vi "Find Downstream Terms.vi"(6 "Distances":dbl[](array[numeric]), 8 "Error":errorcluster, 9 "Segment Descriptors":T1[](array[typedef]) {"Direction" items=["Up", "Down", "Left", "Right"]}, 10 "Terminal Joint Indices":i32[](array[numeric]), 11 "Wire Refnum":refnum<vi>) -> (0 "Error Out":errorcluster, 1 "Array Out":refnum<vi>[](array[refnum]), 2 "Source Node Out":refnum<vi>, 3 "Wire Refnum Out":refnum<vi>)   [LabVIEW 2012, in "Scripting Tools.lvlib"]
doc: "Given an array of wire segment descriptors, an array of terminal joints and an array of distances to an arbitary point, figures out which segment is nearest and then returns all the downstream terminals."
uses:
  Scripting Tools.lvlib
  Wire Segment Descriptor Type.ctl
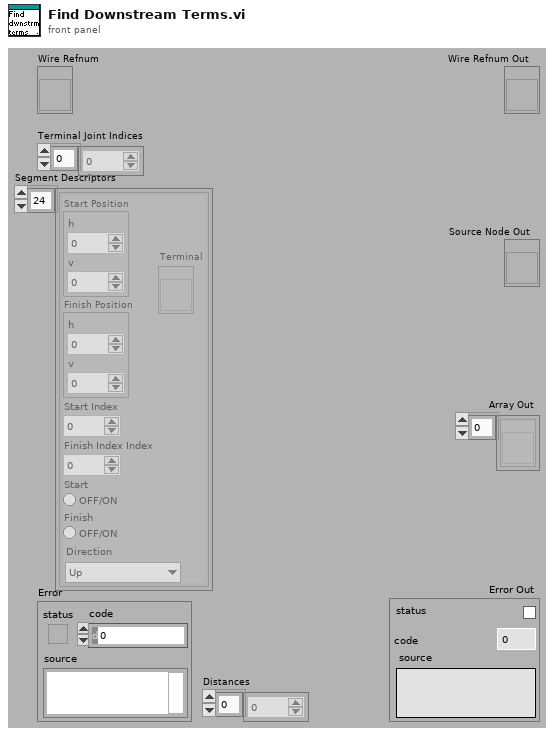
[diagram p1: front panel]
types:
  T1 = typedef "Scripting Tools.lvlib/Wire Segment Descriptor Type.ctl" = cluster{"Start Position":cluster{"h":i16, "v":i16}, "Finish Position":cluster{"h":i16, "v":i16}, "Start Index":i32, "Finish Index Index":i32, "Start":bool, "Finish":bool, "Direction":u16, "Terminal":refnum<vi>}
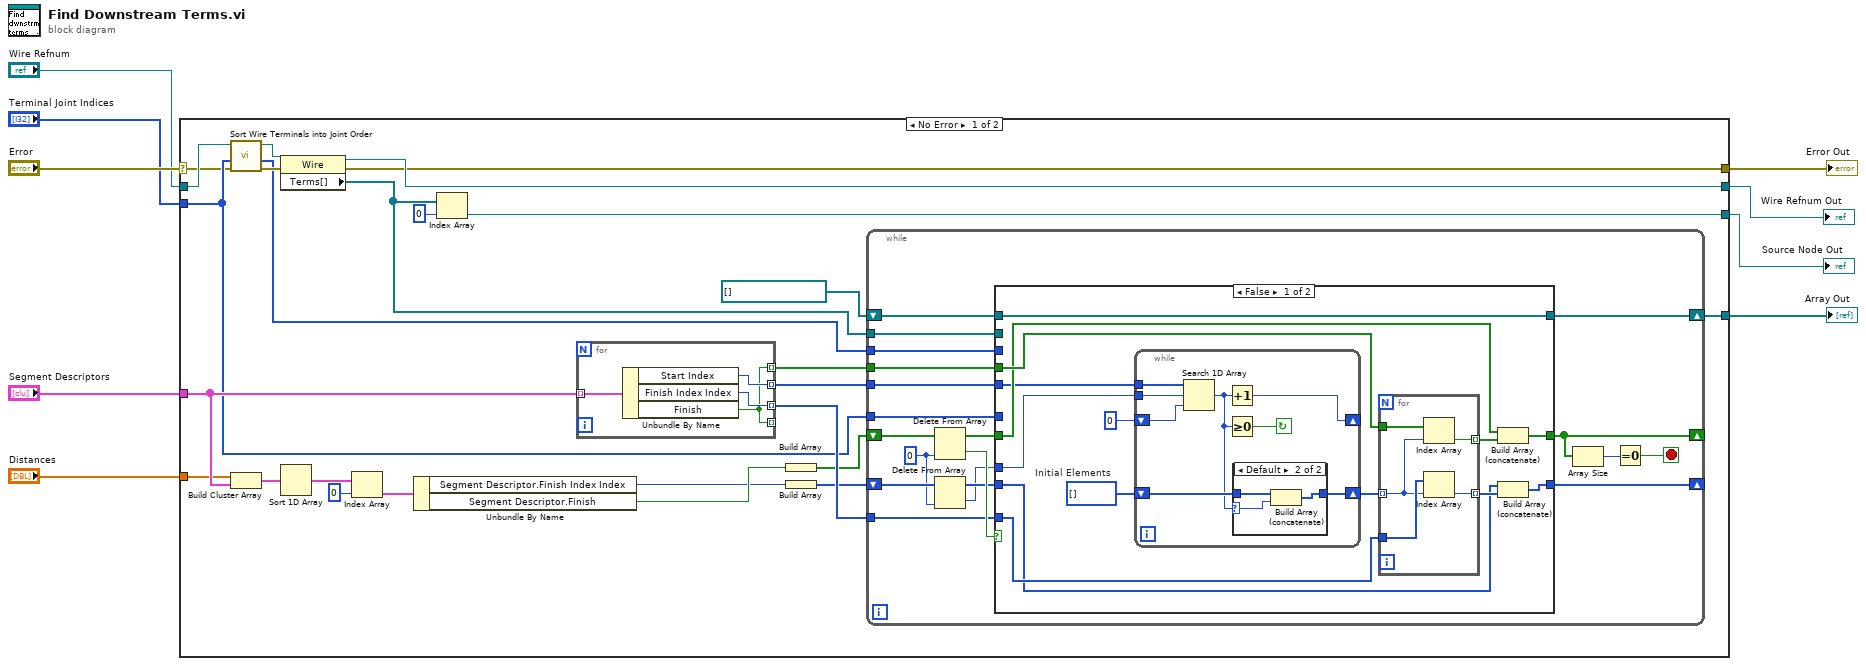
[diagram p0: block diagram]
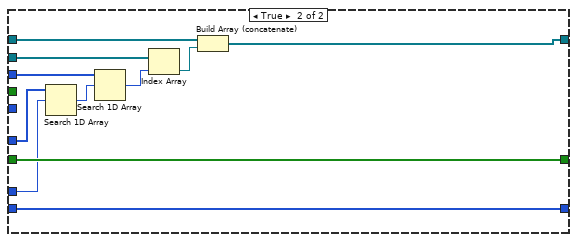
[diagram p3: hidden frame]
diagram:
  n1 = case shown="No Error" "Error" {
    selector: "Error" -> [w10 w102]
    tunnel: [w18 w101] -> w9
    tunnel: [w17 w102] -> w8
    tunnel: "Wire Refnum" -> [w15 w101]
    tunnel: [w34 _] -> w5
    tunnel: [w33 _] -> w4
    tunnel: "Segment Descriptors" -> [w24 _]
    tunnel: "Distances" -> [w19 _]
    tunnel: "Terminal Joint Indices" -> [w12 _]
    frame No Error {
      n2 = call "Sort Wire Terminals into Joint Order.vi"("Error IO"=w10, "Terminal Joint Indices"=w12, "Wire Refnum"=w15) -> ("Error Out"=w13:errorcluster, "Sorted Pointers Out"=w11:i32[], "Wire Refnum Out"=w14:refnum<vi>)  [unwired: 4 in, 2 out]
      n3 = Build Cluster Array(w19, w24) -> (w20:cluster{"d":dbl, "Segment Descriptor":T1}[])
      n4 = property class="Wire"(reference=w14, error in=w13) -> (reference out=w18:refnum<vi>, error out=w17:errorcluster, "Terms[]"=w16:refnum<vi>[])
      n5 = Sort 1D Array(array=w20) -> (sorted array=w21:cluster{"d":dbl, "Segment Descriptor":T1}[])
      n6 = Index Array(array=w21, index=0) -> (element=w23:cluster{"d":dbl, "Segment Descriptor":T1})
      n7 = Unbundle By Name(w23) -> ("Segment Descriptor.Finish Index Index"=w25:i32, "Segment Descriptor.Finish"=w26:bool)
      n8 = Index Array(array=w16, index=0) -> (element=w34:refnum<vi>)
      n9 = for {
        tunnel: w24 -> [w100] mode=indexing
        tunnel: [w99] -> w29 mode=indexing
        tunnel: [w98] -> w30 mode=indexing
        tunnel: [w97] -> _ mode=indexing
        tunnel: [w97] -> w31 mode=indexing
        n10 = Unbundle By Name(w100) -> ("Start Index"=w99:i32, "Finish Index Index"=w98:i32, "Finish"=w97:bool)
      }
      n11 = Build Array(w26) -> (w28:bool[])
      n12 = Build Array(w25) -> (w27:i32[])
      n13 = while {
        shift-right: [w49] -> _
        shift-left: w27 -> [w53]
        shift-right: [w47] -> _
        shift-left: w28 -> [w54]
        tunnel: w29 -> [w44]
        tunnel: w30 -> [w42]
        tunnel: w31 -> [w41]
        tunnel: w11 -> [w40]
        tunnel: w16 -> [w39]
        shift-right: [w38] -> w33
        shift-left: refnum<vi>[] [] -> [w37]
        tunnel: w12 -> [w36]
        stop <- w45 stop-if-true
        w52 = 0 ("index")
        n14 = Delete From Array(array=w54, index=w52) -> (deleted portion=w51:bool, array with subset deleted=w50:bool[])  [unwired: 1 in]
        n15 = Delete From Array(array=w53, index=w52) -> (deleted portion=w43:i32, array with subset deleted=w48:i32[])  [unwired: 1 in]
        n16 = case shown="False" w51 {
          tunnel: [w62 w96] -> w47
          tunnel: w50 -> [w61 w96]
          tunnel: [w65 w95] -> w49
          tunnel: w48 -> [w64 w95]
          tunnel: w44 -> [w56 _]
          tunnel: w43 -> [w57 w87]
          tunnel: w42 -> [w68 _]
          tunnel: w41 -> [w67 _]
          tunnel: w40 -> [_ w94]
          tunnel: w39 -> [_ w92]
          tunnel: [w60 w90] -> w38
          tunnel: w37 -> [w60 w89]
          tunnel: w36 -> [_ w88]
          frame False {
            w59 = i32[] []  # Initial Elements
            n17 = while {
              shift-right: [w69] -> _
              shift-left: 0 ("Start Index (0)") -> [w76]
              shift-right: [w73] -> w55
              shift-left: w59 -> [w74]
              tunnel: w56 -> [w75]
              tunnel: w57 -> [w72]
              stop <- w70 continue-if-true
              n18 = Search 1D Array(1D array=w75, element=w72, start index (0)=w76) -> (index of element=w71:i32)
              n19 = Increment(x=w71) -> (x+1=w69:i32)
              n20 = Greater Or Equal To 0?(x=w71) -> (x >= 0?=w70:bool)
              n21 = case shown="Default" w71 {
                selector: w71 -> [_ w80]
                tunnel: w74 -> [w77 w79]
                tunnel: [w77 w78] -> w73
                frame -1 {
                }
                frame Default {
                  n22 = Build Array (concatenate)(w79, w80) -> (w78:i32[])
                }
              }
            }
            n23 = for {
              tunnel: w68 -> [w85]
              tunnel: w55 -> [w84] mode=indexing
              tunnel: w67 -> [w83]
              tunnel: [w82] -> w66 mode=indexing
              tunnel: [w81] -> w63 mode=indexing
              n24 = Index Array(array=w83, index=w84) -> (element=w81:bool)
              n25 = Index Array(array=w85, index=w84) -> (element=w82:i32)
            }
            n26 = Build Array (concatenate)(w61, w63) -> (w62:bool[])
            n27 = Build Array (concatenate)(w64, w66) -> (w65:i32[])
          }
          frame True {
            n28 = Search 1D Array(1D array=w88, element=w87) -> (index of element=w86:i32)  [unwired: 1 out]
            n29 = Search 1D Array(1D array=w94, element=w86) -> (index of element=w93:i32)  [unwired: 1 out]
            n30 = Index Array(array=w92, index=w93) -> (element=w91:refnum<vi>)
            n31 = Build Array (concatenate)(w89, w91) -> (w90:refnum<vi>[])
          }
        }
        n32 = Array Size(array=w47) -> (size(s)=w46:i32)
        n33 = Equal To 0?(x=w46) -> (x = 0?=w45:bool)
      }
    }
    frame Error {
    }
  }
  "Error Out" <- w8
  "Wire Refnum Out" <- w9
  "Source Node Out" <- w5
  "Array Out" <- w4
